vi "Read LogFile Path.vi"(8 "error in (no error)":errorcluster, 11 "Console Log in":refnum<class "Console Log.lvclass">) -> (0 "error out":errorcluster, 2 "LogFile Path":path, 3 "Console Log out":refnum<class "Console Log.lvclass">)   [LabVIEW 2017, in "Console Log.lvclass"]
uses:
  Console Log.lvclass
  Console Log.lvclass/Console Log.ctl
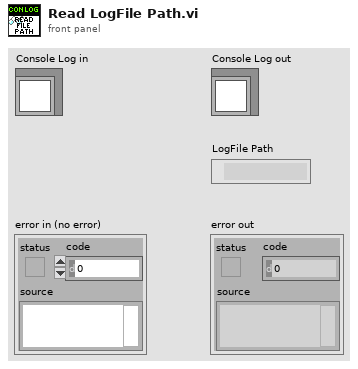
[diagram p1: front panel]
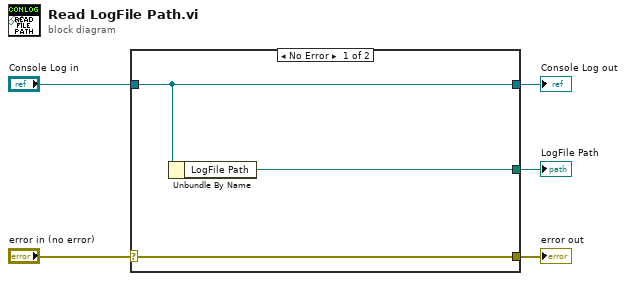
[diagram p0: block diagram]
diagram:
  n1 = case shown="No Error" "error in (no error)" {
    selector: "error in (no error)" -> [w8 w9]
    tunnel: [w8 w9] -> w4
    tunnel: [w7 w10] -> w2
    tunnel: "Console Log in" -> [w7 w10]
    tunnel: [w6 _] -> w1
    frame No Error {
      n2 = Unbundle By Name(w7) -> ("LogFile Path"=w6:path)
    }
    frame Error {
    }
  }
  "error out" <- w4
  "Console Log out" <- w2
  "LogFile Path" <- w1
